vi "Startup.vi"(7 "Application":refnum<class "Application.lvclass">, 8 "error in (no error)":errorcluster, 9 "Config":refnum<class "Config.lvclass">, 10 "DAQ_Engine":refnum<class "DAQ_Engine.lvclass">, 11 "Log_Engine in":refnum<class "Log_Engine.lvclass">) -> (0 "error out":errorcluster, 3 "Log_Engine out":refnum<class "Log_Engine.lvclass">, 5 "Application out":refnum<class "Application.lvclass">)   [LabVIEW 2019, in "Log_Engine.lvclass"]
doc: "Developed by Kevin Thompson\nkevin@thompsonengineering.net\n\nCopyright 2018\nThompson Engineering, LLC"
uses:
  Log_Engine.lvclass
  Config/Config.lvclass
  DAQ_Engine/DAQ_Engine.lvclass
  Application/Application.lvclass
  DataTypes/Dependency--cluster.ctl
  Application/Application.lvclass/Application.ctl
  Config/Config.lvclass/Config.ctl
  Log_Engine.lvclass/Log_Engine.ctl
  Config/Accessors/Get LogEngine Settings.vi
  Application/Accessors/Get InvWfmsQRef.vi
  Accessors/Set Dependency.vi
  Accessors/Set Settings.vi
  Accessors/Set InvWfmsQRef.vi
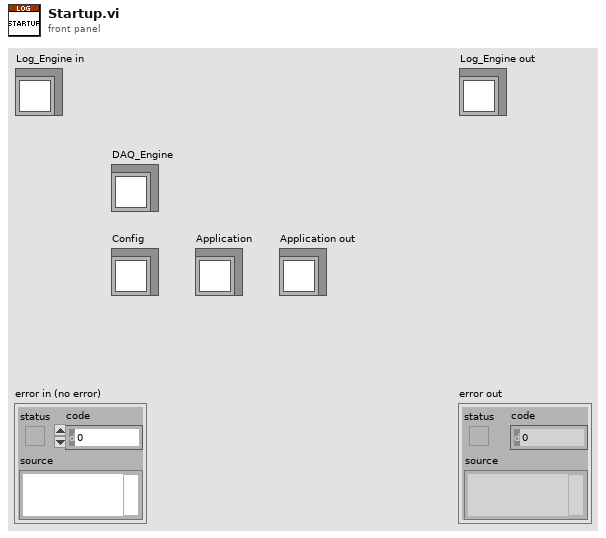
[diagram p1: front panel]
types:
  T1 = typedef "Log_Engine.lvclass/Dependency--cluster.ctl" = cluster{"Config":refnum<class "Config.lvclass">, "DAQ_Engine":refnum<class "DAQ_Engine.lvclass">}
  T2 = typedef "InverterWaveforms--QRef.ctl" = refnum<queue>
  T3 = typedef "Log_Engine.lvclass/Settings--cluster.ctl" = cluster{"Simulation":bool, "TDMS_FolderPath":string, "CSV_FolderPath":string, "TDMS_FileName_Prefix":string, "CSV_FileName_Prefix":string, "TDMS_LogDuration(s)":dbl, "CSV_LogDuration(s)":dbl}
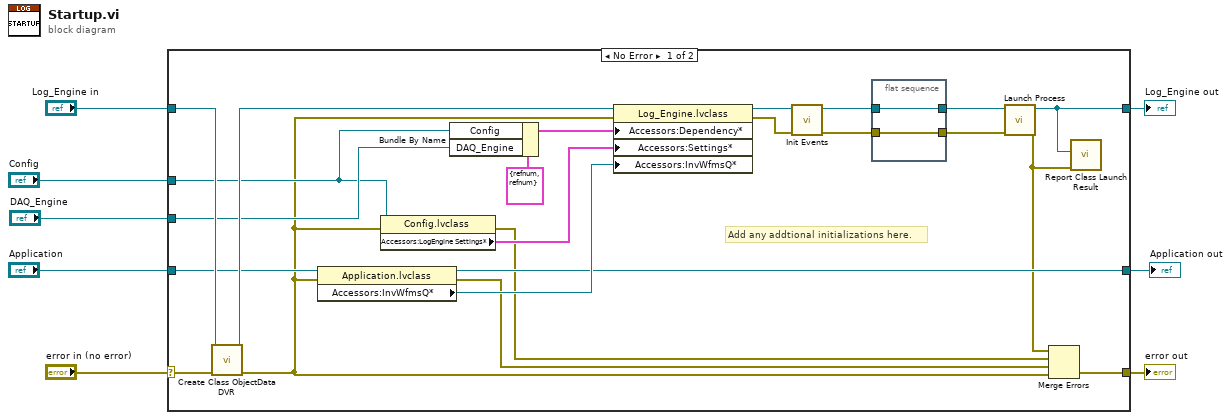
[diagram p0: block diagram]
diagram:
  n1 = case shown="No Error" "error in (no error)" {
    selector: "error in (no error)" -> [w31 w36]
    tunnel: [w24 w36] -> w7
    tunnel: [w15 w35] -> w5
    tunnel: "Log_Engine in" -> [w29 w35]
    tunnel: "Config" -> [w13 _]
    tunnel: "DAQ_Engine" -> [w20 _]
    tunnel: "Application" -> [w19 w34]
    tunnel: [w16 w34] -> w1
    frame No Error {
      # "Add any addtional initializations here."
      n2 = call "Create Class ObjectData DVR.vi"("error in (no error)"=w31, "Log_Engine in"=w29) -> ("error out"=w9:errorcluster, "Log_Engine out"=w28:refnum<class "Log_Engine.lvclass">)  [unwired: 8 in]
      n3 = property class="Application.lvclass"(reference=w19, error in=w9) -> (reference out=w16:refnum<class "Application.lvclass">, error out=w17:errorcluster, "Accessors:InvWfmsQ*"=w18:T2)
      n4 = property class="Config.lvclass"(reference=w13, error in=w9) -> (error out=w10:errorcluster, "Accessors:LogEngine Settings*"=w11:T3)  [unwired: 1 out]
      n5 = Bundle By Name(cluster=T1 {"Config"=refnum, "DAQ_Engine"=refnum} ("Dependency"), "Config"=w13, "DAQ_Engine"=w20) -> (w12:T1)
      n6 = property class="Log_Engine.lvclass"(reference=w28, error in=w9, "Accessors:Dependency*"=w12, "Accessors:Settings*"=w11, "Accessors:InvWfmsQ*"=w18) -> (reference out=w30:refnum<class "Log_Engine.lvclass">, error out=w27:errorcluster)
      n7 = call "Init Events.vi"("error in (no error)"=w27, "Log_Engine in"=w30) -> ("error out"=w25:errorcluster, "Log_Engine out"=w26:refnum<class "Log_Engine.lvclass">)  [unwired: 8 in]
      n8 = flat-sequence {
        tunnel: w26 -> [w33]
        tunnel: [w33] -> w22
        tunnel: w25 -> [w32]
        tunnel: [w32] -> w23
        frame #0 {
        }
      }
      n9 = call "Launch Process.vi"("error in (no error)"=w23, "Log_Engine in"=w22) -> ("error out"=w14:errorcluster, "Log_Engine out"=w15:refnum<class "Log_Engine.lvclass">)  [unwired: 6 in, 2 out]
      n10 = Merge Errors(w14, w10, w17, w9) -> (w24:errorcluster)
      n11 = call "Report Class Launch Result.vi"("Object"=w15, "error in (no error)"=w14) -> ()  [unwired: 8 in, 1 out]
    }
    frame Error {
    }
  }
  "error out" <- w7
  "Log_Engine out" <- w5
  "Application out" <- w1
